vi "BMP085 Close.vi"(8 "error in (no error)":errorcluster, 11 "BMP085 (GY-65) in":refnum<class "BMP085 (GY-65).lvclass">) -> (0 "error out":errorcluster)   [LabVIEW 2015, in "BMP085 (RT).lvlib"]
uses:
  BMP085 (RT).lvlib
  BMP085 (GY-65).lvclass
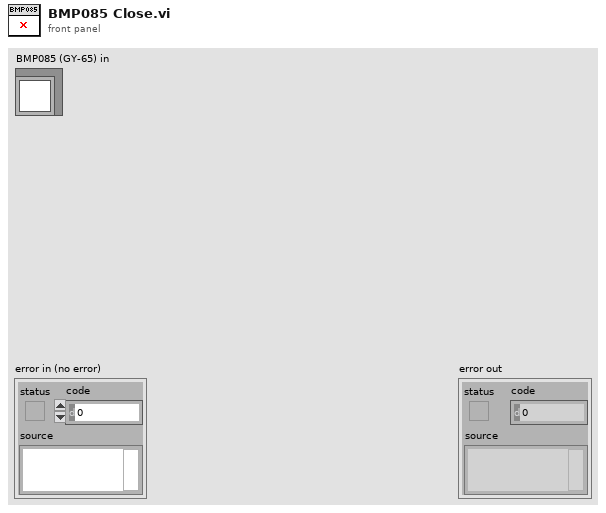
[diagram p1: front panel]
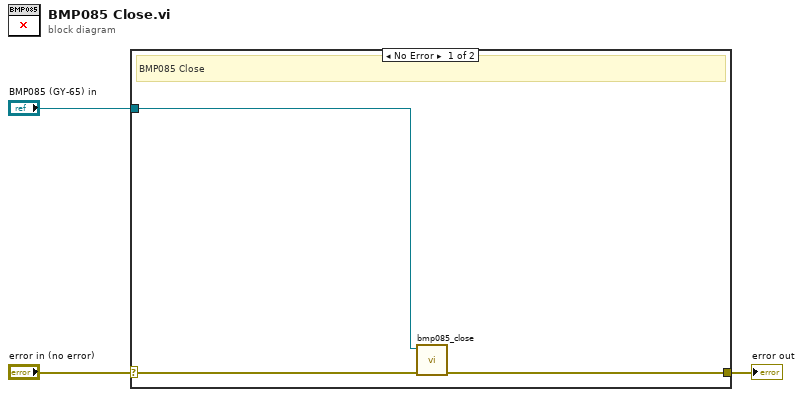
[diagram p0: block diagram]
diagram:
  n1 = case shown="No Error" "error in (no error)" {
    selector: "error in (no error)" -> [w6 w7]
    tunnel: [w5 w7] -> w2
    tunnel: "BMP085 (GY-65) in" -> [w4 _]
    frame No Error {
      # "BMP085 Close"
      n2 = call "bmp085_close.vi"("error in (no error)"=w6, "BMP085 (GY-65) in"=w4) -> ("error out"=w5:errorcluster)  [unwired: 9 in]
    }
    frame Error {
    }
  }
  "error out" <- w2
